vi "Demo1_Service.vi"() -> ()   [LabVIEW 2019]
uses:
  <vilib>/LabVIEW Open Source Project/OpenSerializer JKI JSON/Serializer.JSON.lvclass
  C:/Program Files (x86)/National Instruments/LabVIEW 2019/vi.lib/LabVIEW Open Source Project/OpenSerializer/Serializer/Serializer.lvclass
  <vilib>/LabVIEW Open Source Project/MQTT Connection/MQTT_Base/Base Class/MQTT_Base.lvclass/MQTT_Base.ctl
  <vilib>/LabVIEW Open Source Project/MQTT Client/Client class/Client.lvclass/Client.ctl
  request -- cluster.ctl
  <vilib>/LabVIEW Open Source Project/MQTT Control Packets/Control Packets/ControlPacket/ControlPacket.lvclass/ControlPacket.ctl
  response -- cluster.ctl
  <vilib>/LabVIEW Open Source Project/MQTT TCP Connection/MQTT_TCP/Connection/TCPConnection.lvclass
  C:/Program Files (x86)/National Instruments/LabVIEW 2019/vi.lib/LabVIEW Open Source Project/MQTT Connection/MQTT_Connection/Connection/Connection.lvclass
  <vilib>/LabVIEW Open Source Project/MQTT Client/Client class/Client.lvclass
  C:/Program Files (x86)/National Instruments/LabVIEW 2019/vi.lib/LabVIEW Open Source Project/MQTT Connection/MQTT_Base/Base Class/MQTT_Base.lvclass
  <vilib>/LabVIEW Open Source Project/OpenSerializer/Serializer.FlattenedString/Serializer.FlattenedString.lvclass
  <vilib>/LabVIEW Open Source Project/MQTT Control Packets/Control Packets/PUBLISH/PUBLISH.lvclass
  C:/Program Files (x86)/National Instruments/LabVIEW 2019/vi.lib/LabVIEW Open Source Project/MQTT Control Packets/Control Packets/ControlPacket/ControlPacket.lvclass
  <vilib>/LabVIEW Open Source Project/OpenSerializer/Serializer/Serializer.lvclass
  <vilib>/LabVIEW Open Source Project/MQTT Connection/MQTT_Base/Base Class/MQTT_Base.lvclass
  <vilib>/LabVIEW Open Source Project/OpenSerializer.Base64/Serializer.Base64.lvclass
  <vilib>/LabVIEW Open Source Project/MQTT Control Packets/Control Packets/ControlPacket/ControlPacket.lvclass
panel:
  out "last error":errorcluster
  in  "Connection":bool
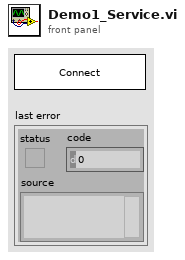
[diagram p1: front panel]
types:
  T1 = typedef "MQTT Client.lvlib/Client.lvclass/Public Events -- cluster.ctl" = cluster{"Connection Status":refnum<user-event>, "Connected":refnum<user-event>, "Application Message":refnum<user-event>}
  T2 = typedef "MQTT Base.lvlib/MQTT_Base.lvclass/Public Events -- cluster.ctl" = cluster{"Stop Event":refnum<user-event>, "Error Event":refnum<user-event>, "Inbound Message":refnum<user-event>}
  T3 = typedef "request -- cluster.ctl" = cluster{"payload":string, "responseURI":string}
  T4 = typedef "response -- cluster.ctl" = cluster{"payload":string, "err-code":i32, "err-msg":string}
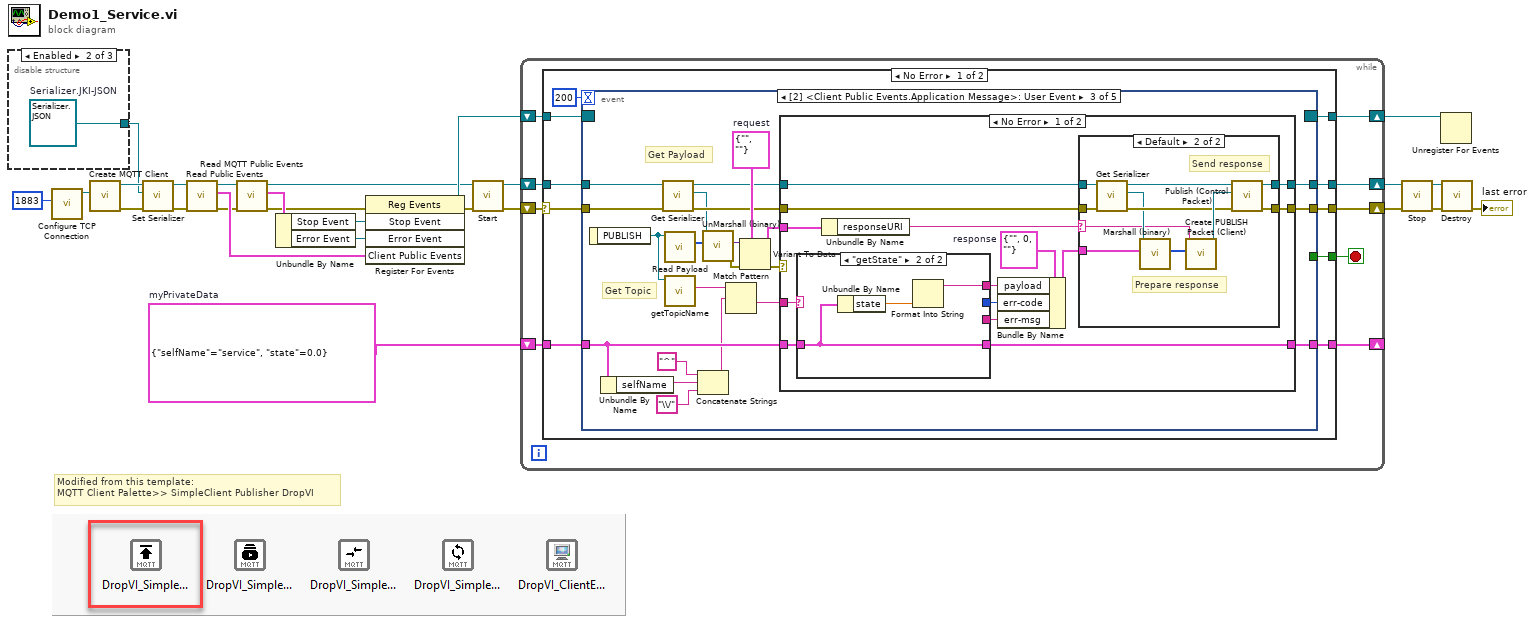
[diagram p0: block diagram]
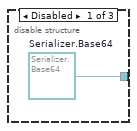
[diagram p2: hidden frame]
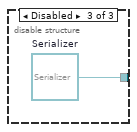
[diagram p3: hidden frame]
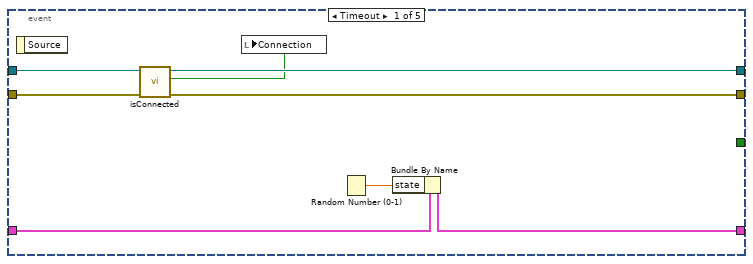
[diagram p4: hidden frame]
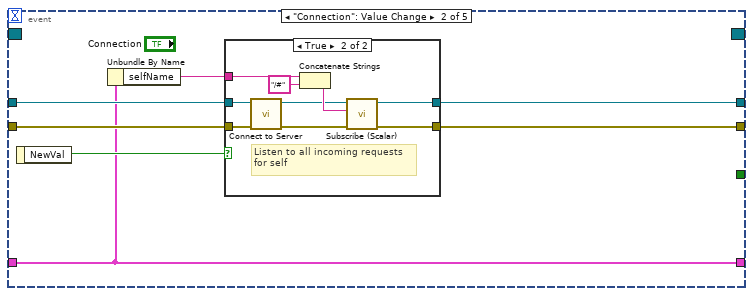
[diagram p5: hidden frame]
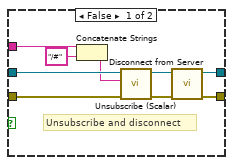
[diagram p6: hidden frame]
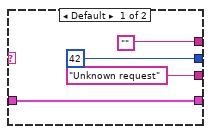
[diagram p8: hidden frame]
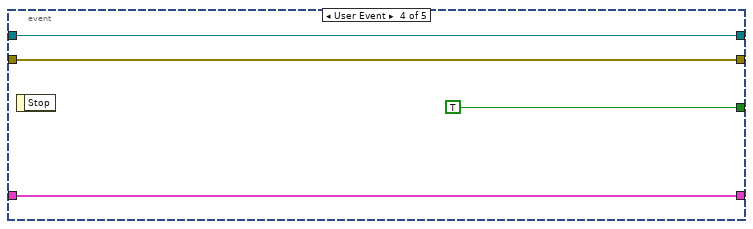
[diagram p10: hidden frame]
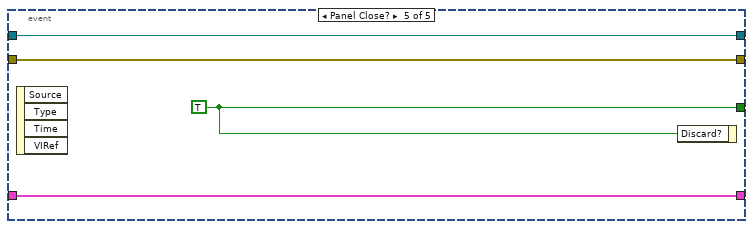
[diagram p11: hidden frame]
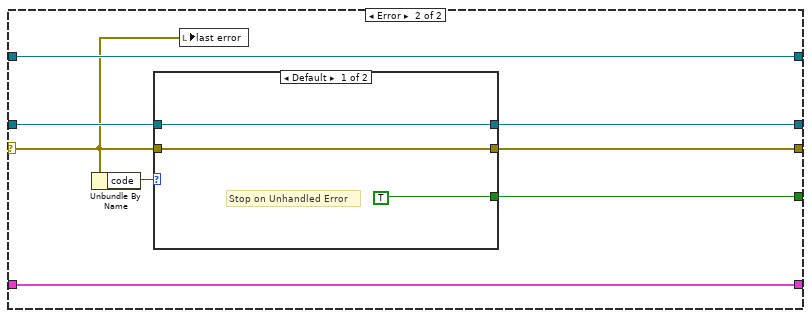
[diagram p12: hidden frame]
diagram:
  w1 = cluster{"selfName":string, "state":dbl} {"selfName"="service", "state"=0.0}  # myPrivateData
  # "Modified from this template:\nMQTT Client Palette>> SimpleClient Publisher DropVI"
  n1 = disable-structure shown="Enabled" {
    disable-tunnel: [w27 w28 w29] -> w2
    frame Disabled {
      w27 = refnum<class "Serializer.Base64.lvclass"> refnum  # Serializer.Base64
    }
    frame Enabled {
      w28 = refnum<class "Serializer.JSON.lvclass"> refnum  # Serializer.JKI-JSON
    }
    frame Disabled {
      w29 = refnum<class "Serializer.lvclass"> refnum  # Serializer
    }
  }
  n2 = call <vilib>:"Configure TCP Connection.vi"("remote port (80)"=u16 1883) -> ("TCPConnection"=w7:refnum<class "TCPConnection.lvclass">)  [unwired: 9 in, 1 out]
  n3 = call <vilib>:"Create MQTT Client.vi"("Connection Configuration"=w7) -> ("error out"=w4:errorcluster, "Client out"=w6:refnum<class "Client.lvclass">)  [unwired: 9 in]
  n4 = call <vilib>:"Set Serializer.vi"("error in (no error)"=w4, "Serializer (default: Flattened String)"=w2, "MQTT_Base"=w6) -> ("error out"=w3:errorcluster, "MQTT_Base out"=w5:refnum<class "Client.lvclass">)  [unwired: 7 in]
  n5 = call <vilib>:"Read Public Events.vi"("error in (no error)"=w3, "Client in"=w5) -> ("error out"=w10:errorcluster, "Client Public Events"=w12:T1, "Client out"=w9:refnum<class "Client.lvclass">)  [unwired: 7 in]
  n6 = call <vilib>:"Read MQTT Public Events.vi"("error in (no error)"=w10, "MQTT_Base in"=w9) -> ("error out"=w11:errorcluster, "MQTT Public Events"=w19:T2, "MQTT_Base out"=w14:refnum<class "Client.lvclass">)  [unwired: 7 in]
  n7 = Unbundle By Name(w19) -> ("Stop Event"=w17:refnum<user-event>, "Error Event"=w18:refnum<user-event>)
  n8 = register-events(error in=w11, w17, w18, w12) -> (reference out=w15:refnum<event-registration>, error out=w13:errorcluster)  [unwired: 1 in]
  n9 = call <vilib>:"Start.vi"("error in (no error)"=w13, "MQTT_Base in"=w14) -> ("error out"=w25:errorcluster, "MQTT_Base out"=w24:refnum<class "Client.lvclass">)  [unwired: 7 in, 1 out]
  n10 = while {
    shift-right: [w37] -> w16
    shift-left: w15 -> [w38]
    shift-right: [w34] -> w21
    shift-left: w24 -> [w35]
    shift-right: [w36] -> w23
    shift-left: w25 -> [w32]
    shift-right: [w31] -> _
    shift-left: w1 -> [w30]
    stop <- w33 stop-if-true
    n11 = case shown="No Error" w32 {
      selector: w32 -> [w41 w150]
      tunnel: w38 -> [w48 w156]
      tunnel: [w47 w156] -> w37
      tunnel: [w46 w152] -> w36
      tunnel: w35 -> [w44 w154]
      tunnel: [w43 w153] -> w34
      tunnel: [w42 w151] -> w33
      tunnel: [w40 w149] -> w31
      tunnel: w30 -> [w39 w149]
      frame No Error {
        n12 = event shown="[2] <Client Public Events.Application Message>: User Event" {
          selector: w48 -> [_ _ _ _ _]
          dyn-events: [_ _ _ _ _] -> w47
          timeout: 200 -> [_ _ _ _ _]
          tunnel: w41 -> [w54 w59 w96 w144 w146]
          tunnel: [w53 w60 w102 w144 w146] -> w46
          tunnel: [_ _ _ TRUE w148] -> w42
          tunnel: w44 -> [w56 w63 w98 w142 w147]
          tunnel: [w55 w61 w103 w142 w147] -> w43
          tunnel: [w52 w58 w90 w141 w145] -> w40
          tunnel: w39 -> [w51 w58 w89 w141 w145]
          event Timeout {
            n13 = event-data() -> ()  [unwired: 1 in, 1 out]
            n14 = call <vilib>:"isConnected.vi"("error in (no error)"=w54, "Client in"=w56) -> ("error out"=w53:errorcluster, "connected"=w49:bool, "Client out"=w55:refnum<class "Client.lvclass">)  [unwired: 7 in]
            n15 = local write "Connection"(w49) -> ()
            n16 = Random Number (0-1)() -> (number: 0 to 1=w50:dbl)
            n17 = Bundle By Name(cluster=w51, "state"=w50) -> (w52:cluster{"selfName":string, "state":dbl})
          }
          event "Connection": Value Change {
            n18 = event-data() -> ("NewVal"=w62:bool)  [unwired: 1 in]
            n19 = Unbundle By Name(w58) -> ("selfName"=w57:string)
            n20 = case shown="True" w62 {
              tunnel: w63 -> [w67 w81]
              tunnel: [w72 w79] -> w61
              tunnel: [w71 w77] -> w60
              tunnel: w59 -> [w65 w80]
              tunnel: w57 -> [w69 w76]
              frame False {
                # "Unsubscribe and disconnect"
                n21 = Concatenate Strings(w69, "/#" ("string")) -> (w64:string)
                n22 = call <vilib>:"Unsubscribe (Scalar).vi"("error in (no error)"=w65, "Topic Filter"=w64, "Client in"=w67) -> ("error out"=w66:errorcluster, "Client out"=w68:refnum<class "Client.lvclass">)  [unwired: 6 in, 1 out]
                n23 = call <vilib>:"Disconnect from Server.vi"("error in (no error)"=w66, "Client in"=w68) -> ("error out"=w71:errorcluster, "Client out"=w72:refnum<class "Client.lvclass">)  [unwired: 7 in, 1 out]
              }
              frame True {
                # "Listen to all incoming requests\nfor self"
                n24 = call <vilib>:"Connect to Server.vi"("error in (no error)"=w80, "Client in"=w81) -> ("error out"=w78:errorcluster, "Client out"=w73:refnum<class "Client.lvclass">)  [unwired: 6 in, 2 out]
                n25 = Concatenate Strings(w76, "/#" ("string")) -> (w74:string)
                n26 = call <vilib>:"Subscribe (Scalar).vi"("error in (no error)"=w78, "Topic Filter"=w74, "Client in"=w73) -> ("error out"=w77:errorcluster, "Client out"=w79:refnum<class "Client.lvclass">)  [unwired: 6 in, 1 out]
              }
            }
          }
          event User Event {
            w101 = T3 {"payload"="", "responseURI"=""}  # request
            # "Get Payload"
            # "Get Topic"
            n27 = event-data() -> ("PUBLISH"=w100:refnum<class "PUBLISH.lvclass">)  [unwired: 1 in]
            n28 = Unbundle By Name(w89) -> ("selfName"=w88:string)
            n29 = call <vilib>:"Get Serializer.vi"("error in (no error)"=w96, "MQTT_Base"=w98) -> ("error out"=w97:errorcluster, "Serializer"=w91:refnum<class "Serializer.lvclass">, "MQTT_Base out"=w99:refnum<class "Client.lvclass">)  [unwired: 7 in]
            n30 = call <vilib>:"Read Payload.vi"("ControlPacket in"=w100) -> ("Payload"=w95:u8[])  [unwired: 9 in, 1 out]
            n31 = call <vilib>:"getTopicName.vi"("PUBLISH in"=w100) -> ("Topic"=w84:string)  [unwired: 8 in, 2 out]
            n32 = Concatenate Strings("^" ("string"), w88, "\\/" ("string")) -> (w85:string)
            n33 = call <vilib>:"UnMarshall (binary).vi"("Bytes"=w95, "Serializer in"=w91) -> ("error out"=w82:errorcluster, "Variant"=w94:variant)  [unwired: 7 in, 1 out]
            n34 = Match Pattern(string=w84, regular expression=w85) -> (after substring=w83:string)  [unwired: 1 in, 3 out]
            n35 = Variant To Data(error in=w82, type=w101, Variant=w94) -> (data=w92:T3, error out=w93:errorcluster)
            n36 = case shown="No Error" w93 {
              tunnel: [w117 w140] -> w103
              tunnel: [w116 w139] -> w102
              tunnel: w92 -> [w114 _]
              tunnel: w83 -> [w115 _]
              tunnel: w99 -> [w112 w140]
              tunnel: w97 -> [w113 w139]
              tunnel: [w107 w138] -> w90
              tunnel: w89 -> [w106 w138]
              frame No Error {
                w111 = T4 {"payload"="", "err-code"=0, "err-msg"=""}  # response
                n37 = case shown="\"getState\"" w115 {
                  tunnel: [42 _] -> w109
                  tunnel: ["Unknown request" ("err-msg") _] -> w108
                  tunnel: [w132 w137] -> w107
                  tunnel: w106 -> [w132 w137]
                  tunnel: ["" w135] -> w105
                  frame Default {
                  }
                  frame "getState" {
                    n38 = Unbundle By Name(w137) -> ("state"=w136:dbl)
                    n39 = Format Into String(w136) -> (resulting string=w135:string)  [unwired: 3 in, 1 out]
                  }
                }
                n40 = Unbundle By Name(w114) -> ("responseURI"=w104:string)
                n41 = Bundle By Name(cluster=w111, "payload"=w105, "err-code"=w109, "err-msg"=w108) -> (w110:T4)
                n42 = case shown="Default" w104 {
                  selector: w104 -> [_ w120]
                  tunnel: [w119 w130] -> w117
                  tunnel: [w118 w129] -> w116
                  tunnel: w113 -> [w118 w125]
                  tunnel: w112 -> [w119 w123]
                  tunnel: w110 -> [_ w121]
                  frame "\u0000" {
                    # "no response URI"
                  }
                  frame Default {
                    # "Prepare response"
                    # "Send response"
                    n43 = call <vilib>:"Get Serializer.vi"("error in (no error)"=w125, "MQTT_Base"=w123) -> ("error out"=w126:errorcluster, "Serializer"=w122:refnum<class "Serializer.lvclass">, "MQTT_Base out"=w124:refnum<class "Client.lvclass">)  [unwired: 7 in]
                    n44 = call <vilib>:"Marshall (binary).vi"("Variant"=w121, "Serializer in"=w122) -> ("Bytes"=w127:u8[])  [unwired: 7 in, 2 out]
                    n45 = call <vilib>:"Create PUBLISH Packet (Client).vi"("Payload"=w127, "Topic Name"=w120) -> ("PUBLISH"=w128:refnum<class "PUBLISH.lvclass">)  [unwired: 6 in, 3 out]
                    n46 = call <vilib>:"Publish (Control Packet).vi"("error in (no error)"=w126, "PUBLISH"=w128, "Client in"=w124) -> ("error out"=w129:errorcluster, "Client out"=w130:refnum<class "Client.lvclass">)  [unwired: 6 in, 1 out]
                  }
                }
              }
              frame Error {
                # "Invalid Packet Format.\nReject request. No response possible."
              }
            }
          }
          event User Event {
            n47 = event-data() -> ()  [unwired: 1 in, 1 out]
          }
          event Panel Close? {
            w148 = TRUE
            n48 = event-data() -> ()  [unwired: 1 in, 4 out]
            n49 = event-data("Discard?"=w148) -> ()  [unwired: 1 in, 1 out]
          }
        }
      }
      frame Error {
        n50 = Unbundle By Name(w150) -> ("code"=w155:i32)
        n51 = case shown="Default" w155 {
          tunnel: w154 -> [w159 w160]
          tunnel: [w159 w160] -> w153
          tunnel: w150 -> [w158 _]
          tunnel: [w158 _] -> w152
          tunnel: [TRUE _] -> w151
          frame Default {
            # "Stop on Unhandled Error"
          }
          frame 56, 63, 66 {
            # "Disconnected"
          }
        }
        n52 = local write "last error"(w150) -> ()
      }
    }
  }
  n53 = call <vilib>:"Stop.vi"("error in (no error)"=w23, "MQTT_Base in"=w21) -> ("error out"=w22:errorcluster, "MQTT_Base out"=w20:refnum<class "Client.lvclass">)  [unwired: 7 in, 1 out]
  n54 = Unregister For Events(event registration refnum=w16) -> ()  [unwired: 1 in, 1 out]
  n55 = call <vilib>:"Destroy.vi"("error in (no error)"=w22, "MQTT_Base in"=w20) -> ("error out"=→"last error":errorcluster)  [unwired: 8 in, 1 out]
